vi "CoMP-S Rotation and Focus Check.vi"() -> (1 "OBS_PROG OUT":string, 2 "Observer OUT":string)   [LabVIEW 2014]
panel:
  in  "Observer Programm":u16(ring) items=["Unknown", "TEST", "OBS_PROG 001: SPEKTROPOLARIMETRIA POKOJNEJ PROTUBERANCIE A JEJ KAVITY - 854,656,637,530 (P.Schwartz)", "OBS_PROG 002: SPEKTROPOLARIMETRIA POKOJNEJ PROTUBERANCIE - 656 (Y.Su)", "OBS_PROG 003: SPEKTROPOLARIMETRIA PROTUBERANCII A KORONY - 656,587,530 (P.Schwartz)", "OBS_PROG 004: SPEKTROPOLARIMETRIA FILAMENTOV NA DISKU - 854,656,587 (P.Schwartz)", "OBS_PROG 005: SPEKTROPOLARIMETRIA PROTUBERANCII -s 854,656,587,530 (P.Schwartz)", "OBS_PROG 006: SPEKTROPOLARIMETRIA PROTUBERANCII A KORONY - 854,656,587,530 (P.Schwartz)", "CAL_PROG 001: CORONAGRAPH FOCUS DETERMINATION FOR ALL LINES", "TEST_PROG 001: DATA ACQUISITION BY CAMERAS"]
  in  "Observer":u16(ring) items=["Unknown", "AMBROZ", "HABAJ", "KAVKA", "KOZAK", "MACURA", "RYBAK", "INY"]
  out "New Diffuser Status":string
  in  "file path (use dialog) 3":path=path "C:/CoMP-S Observer/diffuser.txt"
  in  "Set Diffueser Status":u16(ring)=1 items=["OUT OF BEAM (OPEN)", "IN BEAM (CLOSED)"]
  out "Diffuser Status":string
  in  "Set Rotation Angle":dbl
  in  "Set Focus":dbl=103.0 format="%.1f"
  out "New Rotation":ext
  out "New Focus":ext
  out "Focus":ext
  in  "file path (use dialog) 2":path=path "C:/CoMP-S OBSERVER/focus.txt"
  in  "stop":bool
  out "Rotation angle":ext
  in  "file path (use dialog)":path=path "C:/CoMP-S OBSERVER/rotation.txt"
  # "Please check default values of CoMP-S position anle, \ncoronagraph focus, and\ndiffuser status !!!"
  # "If values are right, then press OK"
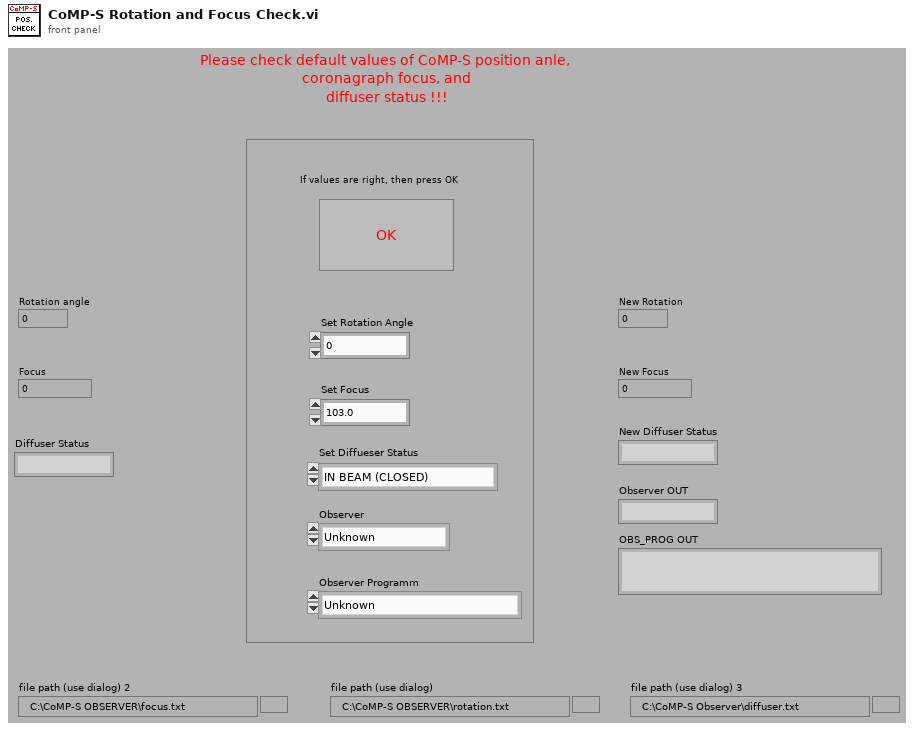
[diagram p1: front panel]
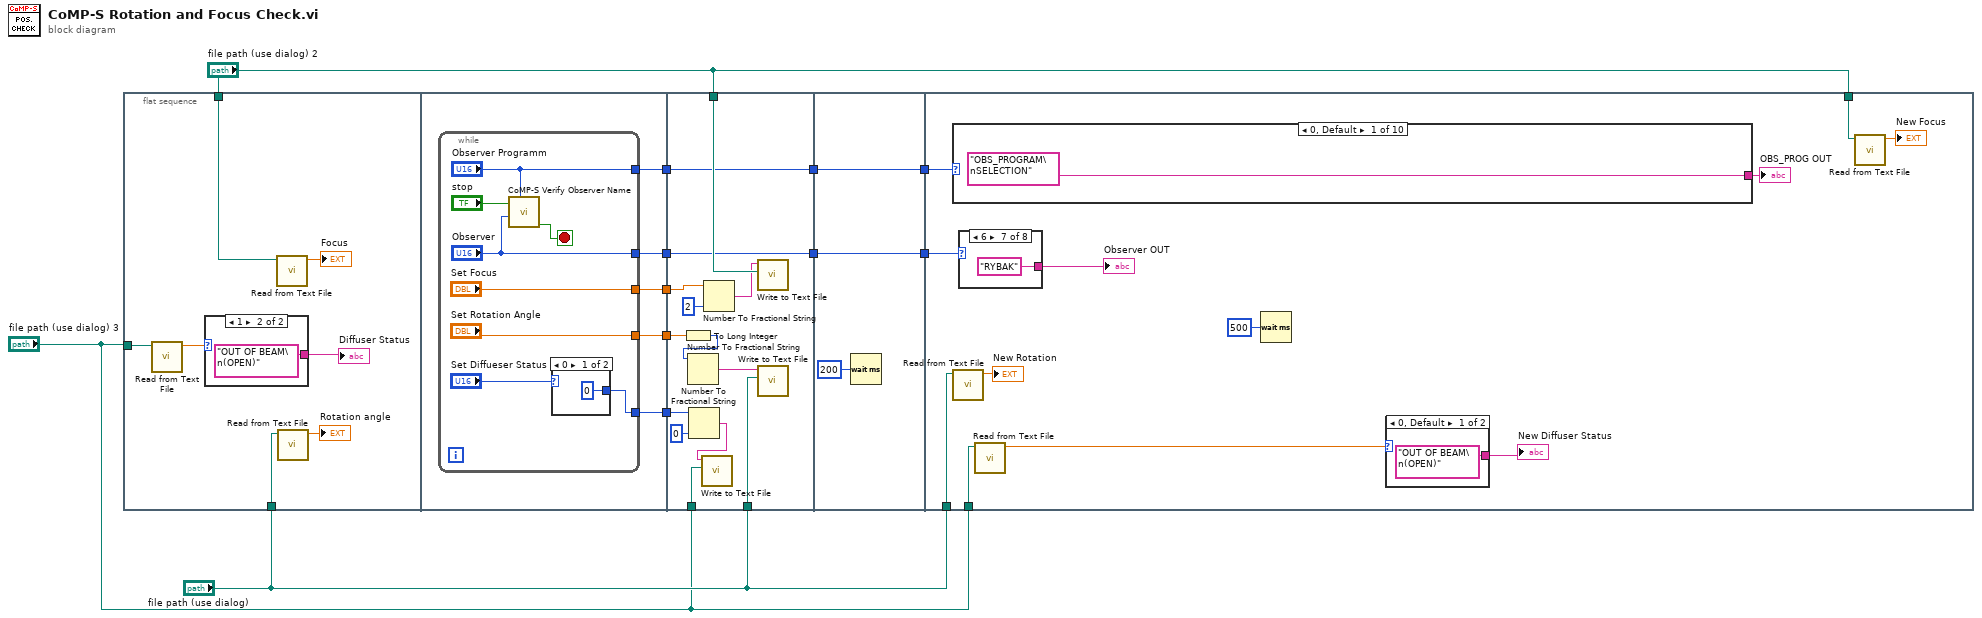
[diagram p0: block diagram]
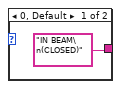
[diagram p2: hidden frame]
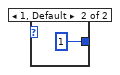
[diagram p3: hidden frame]
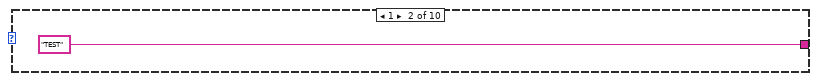
[diagram p4: hidden frame]
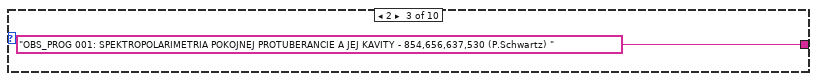
[diagram p5: hidden frame]
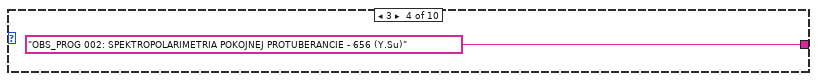
[diagram p6: hidden frame]
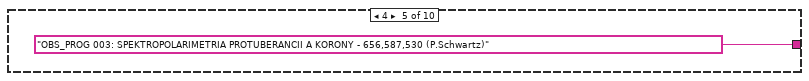
[diagram p7: hidden frame]
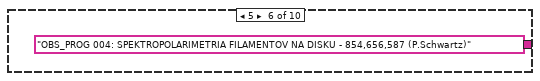
[diagram p8: hidden frame]
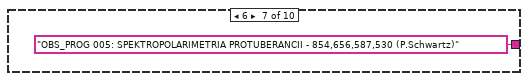
[diagram p9: hidden frame]
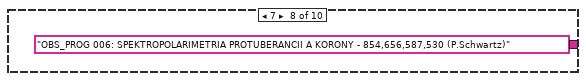
[diagram p10: hidden frame]
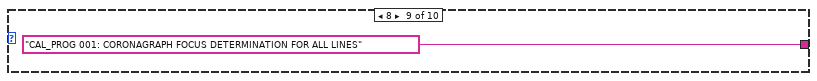
[diagram p11: hidden frame]
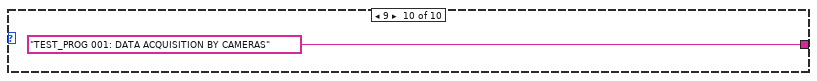
[diagram p12: hidden frame]
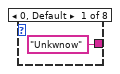
[diagram p13: hidden frame]
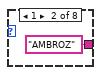
[diagram p14: hidden frame]
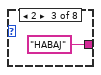
[diagram p15: hidden frame]
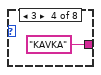
[diagram p16: hidden frame]
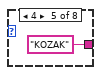
[diagram p17: hidden frame]
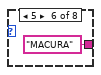
[diagram p18: hidden frame]
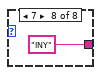
[diagram p19: hidden frame]
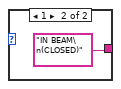
[diagram p20: hidden frame]
diagram:
  n1 = flat-sequence {
    tunnel: "file path (use dialog) 2" -> [w17]
    tunnel: "file path (use dialog)" -> [w16]
    tunnel: "file path (use dialog) 3" -> [w13]
    tunnel: [w26] -> w12
    tunnel: [w25] -> w11
    tunnel: [w24] -> w8
    tunnel: [w23] -> w4
    tunnel: [w22] -> w3
    tunnel: w12 -> [w47]
    tunnel: w11 -> [w45]
    tunnel: "file path (use dialog)" -> [w50]
    tunnel: "file path (use dialog) 2" -> [w49]
    tunnel: w8 -> [w42]
    tunnel: "file path (use dialog) 3" -> [w39]
    tunnel: [w38] -> w5
    tunnel: w4 -> [w38]
    tunnel: w3 -> [w37]
    tunnel: [w37] -> w2
    tunnel: [w52] -> w6
    tunnel: w5 -> [w52]
    tunnel: w2 -> [w51]
    tunnel: [w51] -> w1
    tunnel: "file path (use dialog) 2" -> [w63]
    tunnel: "file path (use dialog)" -> [w62]
    tunnel: "file path (use dialog) 3" -> [w60]
    tunnel: w6 -> [w57]
    tunnel: w1 -> [w54]
    frame #0 {
      n2 = call "Read from Text File.vi"("file path (use dialog)"=w13) -> ("number"=w15:ext)  [unwired: 8 in, 2 out]
      n3 = case shown="1" w15 {
        tunnel: ["IN BEAM\n(CLOSED)" "OUT OF BEAM\n(OPEN)"] -> w14
        frame 0, Default {
        }
        frame 1 {
        }
      }
      "Diffuser Status" <- w14
      n4 = call "Read from Text File.vi"("file path (use dialog)"=w17) -> ("number"=→"Focus":ext)  [unwired: 8 in, 2 out]
      n5 = call "Read from Text File.vi"("file path (use dialog)"=w16) -> ("number"=→"Rotation angle":ext)  [unwired: 8 in, 2 out]
    }
    frame #1 {
      n6 = while {
        tunnel: ["Set Focus"] -> w26
        tunnel: ["Set Rotation Angle"] -> w25
        tunnel: [w31] -> w24
        tunnel: ["Observer"] -> w23
        tunnel: ["Observer Programm"] -> w22
        stop <- w28 stop-if-true
        n7 = call "CoMP-S Verify Observer Name.vi"("Observer Programm"="Observer Programm", "Observer 2"="Observer", "Stop Button"="stop") -> ("Out Stop"=w28:bool)  [unwired: 6 in, 2 out]
        n8 = case shown="0" "Set Diffueser Status" {
          tunnel: [0 1] -> w31
          frame 0 {
          }
          frame 1, Default {
          }
        }
      }
    }
    frame #2 {
      n9 = To Long Integer(number=w45) -> (32bit integer=w44:i32)
      n10 = Number To Fractional String(number=w44) -> (F-format string=w43:string)  [unwired: 3 in]
      n11 = Number To Fractional String(number=w42, precision (6)=i16 0) -> (F-format string=w41:string)  [unwired: 2 in]
      n12 = call "Write to Text File.vi"("file path (use dialog)"=w39, "text"=w41) -> ()  [unwired: 9 in, 1 out]
      n13 = Number To Fractional String(number=w47, precision (6)=i16 2) -> (F-format string=w48:string)  [unwired: 2 in]
      n14 = call "Write to Text File.vi"("file path (use dialog)"=w49, "text"=w48) -> ()  [unwired: 9 in, 1 out]
      n15 = call "Write to Text File.vi"("file path (use dialog)"=w50, "text"=w43) -> ()  [unwired: 9 in, 1 out]
    }
    frame #3 {
      n16 = Wait (ms)(milliseconds to wait=u32 200) -> ()  [unwired: 1 out]
    }
    frame #4 {
      n17 = case shown="0, Default" w54 {
        tunnel: ["OBS_PROGRAM\nSELECTION" "TEST" "OBS_PROG 001: SPEKTROPOLARIMETRIA POKOJNEJ PROTUBERANCIE A JEJ KAVITY - 854,656,637,530 (P.Schwartz) " "OBS_PROG 002: SPEKTROPOLARIMETRIA POKOJNEJ PROTUBERANCIE - 656 (Y.Su)" "OBS_PROG 003: SPEKTROPOLARIMETRIA PROTUBERANCII A KORONY - 656,587,530 (P.Schwartz)" "OBS_PROG 004: SPEKTROPOLARIMETRIA FILAMENTOV NA DISKU - 854,656,587 (P.Schwartz)" "OBS_PROG 005: SPEKTROPOLARIMETRIA PROTUBERANCII - 854,656,587,530 (P.Schwartz)" "OBS_PROG 006: SPEKTROPOLARIMETRIA PROTUBERANCII A KORONY - 854,656,587,530 (P.Schwartz)" "CAL_PROG 001: CORONAGRAPH FOCUS DETERMINATION FOR ALL LINES" "TEST_PROG 001: DATA ACQUISITION BY CAMERAS"] -> w55
        frame 0, Default {
        }
        frame 1 {
        }
        frame 2 {
        }
        frame 3 {
        }
        frame 4 {
        }
        frame 5 {
        }
        frame 6 {
        }
        frame 7 {
        }
        frame 8 {
        }
        frame 9 {
        }
      }
      "OBS_PROG OUT" <- w55
      n18 = call "Read from Text File.vi"("file path (use dialog)"=w62) -> ("number"=→"New Rotation":ext)  [unwired: 8 in, 2 out]
      n19 = case shown="6" w57 {
        tunnel: ["Unkwnow" "AMBROZ" "HABAJ" "KAVKA" "KOZAK" "MACURA" "RYBAK" "INY"] -> w56
        frame 0, Default {
        }
        frame 1 {
        }
        frame 2 {
        }
        frame 3 {
        }
        frame 4 {
        }
        frame 5 {
        }
        frame 6 {
        }
        frame 7 {
        }
      }
      "Observer OUT" <- w56
      n20 = call "Read from Text File.vi"("file path (use dialog)"=w60) -> ("number"=w58:ext)  [unwired: 8 in, 2 out]
      n21 = Wait (ms)(milliseconds to wait=u32 500) -> ()  [unwired: 1 out]
      n22 = case shown="0, Default" w58 {
        tunnel: ["OUT OF BEAM\n(OPEN)" "IN BEAM\n(CLOSED)"] -> w59
        frame 0, Default {
        }
        frame 1 {
        }
      }
      "New Diffuser Status" <- w59
      n23 = call "Read from Text File.vi"("file path (use dialog)"=w63) -> ("number"=→"New Focus":ext)  [unwired: 8 in, 2 out]
    }
  }
